vi "test Log Span Time.vi"(8 "error in":errorcluster, 11 "TestCase in":refnum<class "Embedded Data Logger Windows System Tests.lvclass">) -> (0 "error out":errorcluster, 3 "TestCase out":refnum<class "Embedded Data Logger Windows System Tests.lvclass">)   [LabVIEW 2027, in "Embedded Data Logger Windows System Tests.lvclass"]
uses:
  Embedded Data Logger Windows System Tests.lvclass
  3b46ef18-90ca-459a-b563-5d08ad5bcdeb.vi
  7aa6e89f-c275-46aa-8aa6-7be364725cbe.vi
  150ac966-a804-44a1-88cd-42a06859b817.vi
  C:/Program Files/National Instruments/LabVIEW 2027/vi.lib/addons/_JKI Toolkits/VI Tester/TestCase.llb/TestCase.lvclass
  <vilib>/addons/_JKI Toolkits/VI Tester/TestCase.llb/TestCase.lvclass
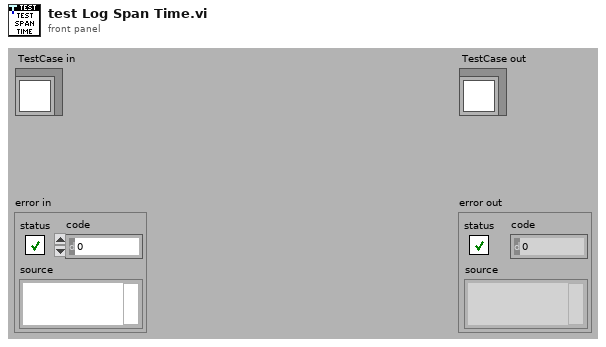
[diagram p1: front panel]
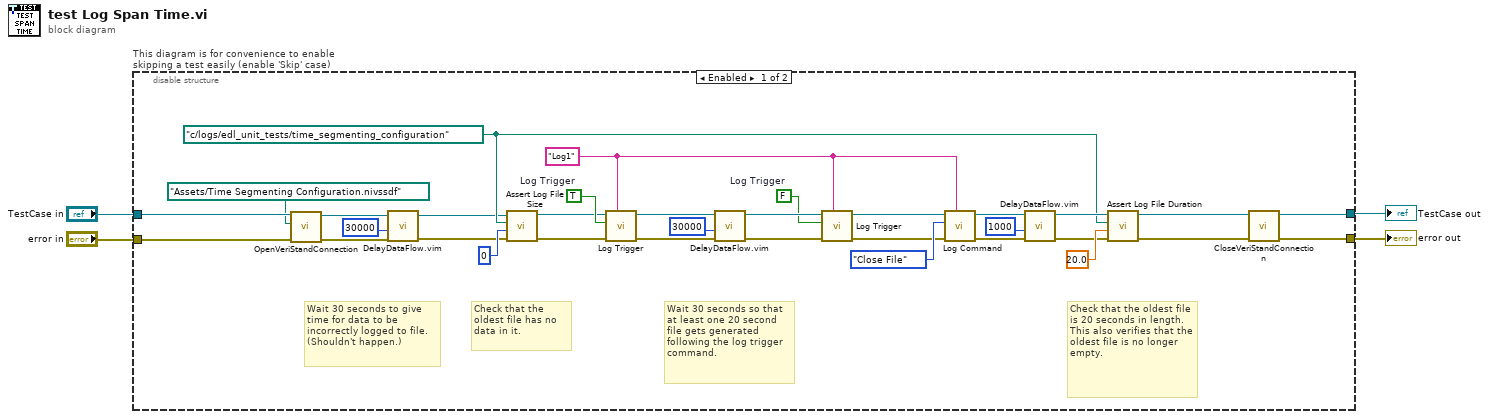
[diagram p0: block diagram]
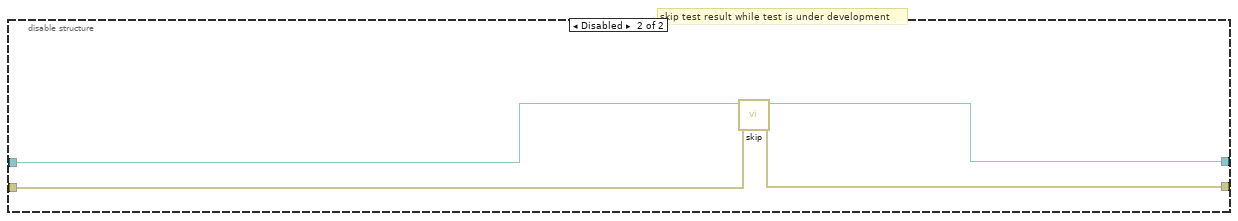
[diagram p2: hidden frame]
diagram:
  n1 = disable-structure "This diagram is for convenience to enable skipping a test easily (enable 'Skip' case)" shown="Enabled" {
    disable-tunnel: "TestCase in" -> [w20 w37]
    disable-tunnel: [w16 w35] -> w1
    disable-tunnel: [w17 w36] -> w3
    disable-tunnel: "error in" -> [w21 w34]
    frame Enabled {
      w22 = path "c:/logs/edl_unit_tests/time_segmenting_configuration" ("file path")
      w26 = "Log1" ("Embedded Data Logger File Name")
      w32 = FALSE  # Log Trigger
      w31 = TRUE  # Log Trigger
      # "Check that the oldest file has no data in it."
      # "Wait 30 seconds to give time for data to be incorrectly logged to file. (Shouldn't happen.)"
      # "Check that the oldest file is 20 seconds in length.\nThis also verifies that the oldest file is no longer empty."
      # "Wait 30 seconds so that at least one 20 second file gets generated following the log trigger command."
      n2 = call-dynamic "OpenVeriStandConnection.vi"("error in (no error)"=w21, "System Definition File"=path "Assets/Time Segmenting Configuration.nivssdf", "VeriStand Test Case in"=w20) -> ("error out"=w12:errorcluster, "VeriStand Test Case out"=w19:refnum<class "Embedded Data Logger Windows System Tests.lvclass">)  [unwired: 6 in, 1 out]
      n3 = call "DelayDataFlow.vim"("value in"=w12, "milliseconds to wait"=u32 30000) -> ("value out"=w11:errorcluster)  [unwired: 2 in, 1 out]
      n4 = call "Assert Log File Size.vi"("Expected size of file in bytes"=i64 0, "file path"=w22, "Embedded Data Logger System Tests in"=w19) -> ("Embedded Data Logger System Tests out"=w25:refnum<class "Embedded Data Logger Windows System Tests.lvclass">)  [unwired: 7 in, 1 out]
      n5 = call "Log Trigger.vi"("Embedded Data Logger File Name"=w26, "error in"=w11, "Log Trigger"=w31, "Embedded Data Logger System Tests in"=w25) -> ("error out"=w9:errorcluster, "Embedded Data Logger System Tests out"=w33:refnum<class "Embedded Data Logger Windows System Tests.lvclass">)  [unwired: 6 in]
      n6 = call "DelayDataFlow.vim"("value in"=w9, "milliseconds to wait"=u32 30000) -> ("value out"=w8:errorcluster)  [unwired: 2 in, 1 out]
      n7 = call "Log Trigger.vi"("Embedded Data Logger File Name"=w26, "error in"=w8, "Log Trigger"=w32, "Embedded Data Logger System Tests in"=w33) -> ("error out"=w29:errorcluster, "Embedded Data Logger System Tests out"=w28:refnum<class "Embedded Data Logger Windows System Tests.lvclass">)  [unwired: 6 in]
      n8 = call "Log Command.vi"("Embedded Data Logger File Name"=w26, "error in"=w29, "Log Command"=enum16{"Idle", "Open File", "Close File"}."Close File", "Embedded Data Logger System Tests in"=w28) -> ("error out"=w6:errorcluster, "Embedded Data Logger System Tests out"=w27:refnum<class "Embedded Data Logger Windows System Tests.lvclass">)  [unwired: 6 in]
      n9 = call "DelayDataFlow.vim"("value in"=w6, "milliseconds to wait"=u32 1000) -> ("value out"=w5:errorcluster)  [unwired: 2 in, 1 out]
      n10 = call "Assert Log File Duration.vi"("error in"=w5, "Expected file duration (s)"=20.0, "File Directory"=w22, "Embedded Data Logger System Tests in"=w27) -> ("error out"=w18:errorcluster, "Embedded Data Logger System Tests out"=w15:refnum<class "Embedded Data Logger Windows System Tests.lvclass">)  [unwired: 6 in]
      n11 = call-dynamic "CloseVeriStandConnection.vi"("error in (no error)"=w18, "VeriStand Test Case in"=w15) -> ("error out"=w17:errorcluster, "VeriStand Test Case out"=w16:refnum<class "Embedded Data Logger Windows System Tests.lvclass">)  [unwired: 8 in]
    }
    frame Disabled {
      # "skip test result while test is under development"
      n12 = call <vilib>:"skip.vi"("error in (no error)"=w34, "TestCase in"=w37) -> ("error out"=w36:errorcluster, "TestCase out"=w35:refnum<class "Embedded Data Logger Windows System Tests.lvclass">)  [unwired: 8 in]
    }
  }
  "error out" <- w3
  "TestCase out" <- w1
